vi "GetChimeraResources.vi"(8 "error in (no error)":errorcluster, 11 "Automotive Vision Device selector":refnum<vi>) -> (0 "error out":errorcluster, 1 "Bitfiles":string[](array[string]), 2 "Available input channels on Automotive Camera Vision Devices":string[][](array[string]), 3 "Device Aliases":string[](array[string]))   [LabVIEW 2025]
doc: "Finds all available Automative Vision devices (like PXIe-1486, etc.) , filter them for those what has inputs, gathers all of the input channels, resources, types, and corresponding bitfile."
uses:
  <vilib>/nisyscfg/Filter Mode.ctl
  <vilib>/nisyscfg/nisyscfg.lvlib
  <resource>/objmgr/niflexrioatomicsae.rc
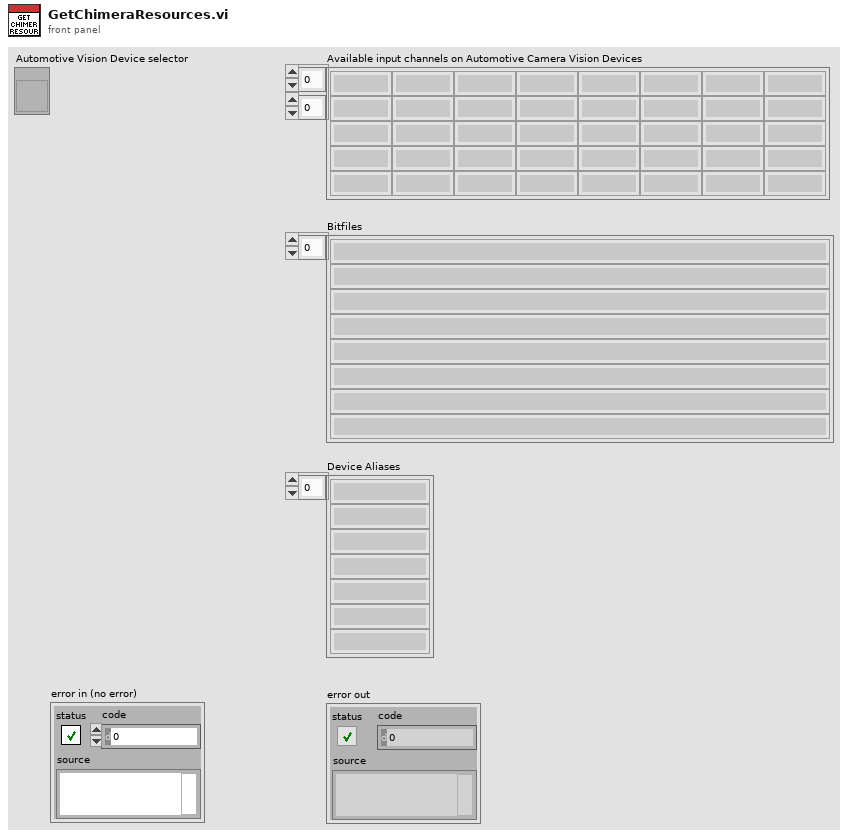
[diagram p1: front panel]
types:
  T1 = typedef "nisyscfg.lvlib/Filter Mode.ctl" = i32
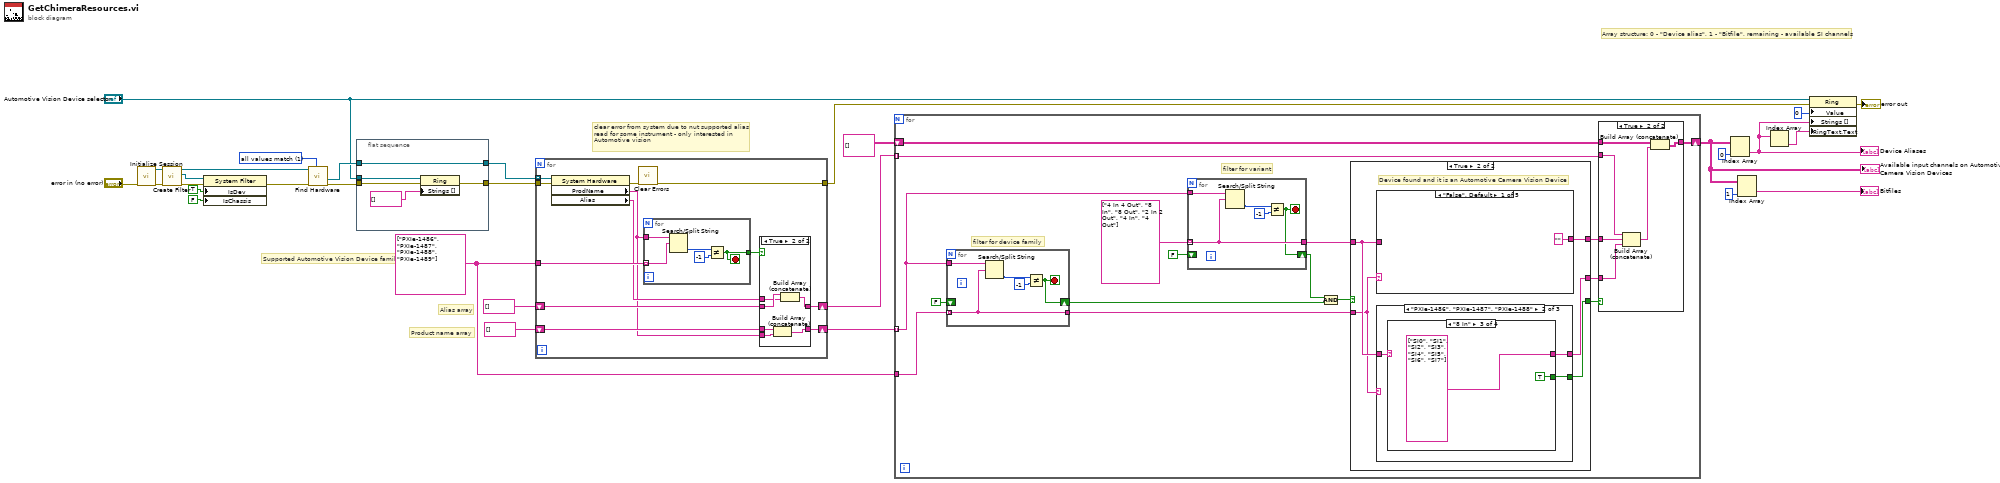
[diagram p0: block diagram]
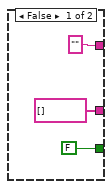
[diagram p3: hidden frame]
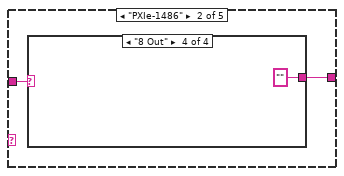
[diagram p4: hidden frame]
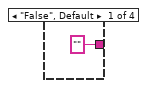
[diagram p5: hidden frame]
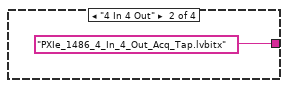
[diagram p6: hidden frame]
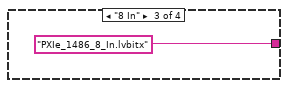
[diagram p7: hidden frame]
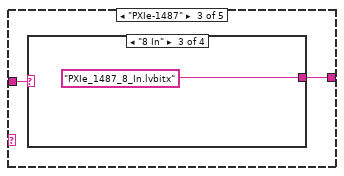
[diagram p8: hidden frame]
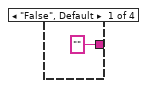
[diagram p9: hidden frame]
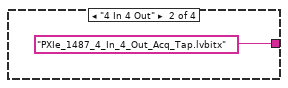
[diagram p10: hidden frame]
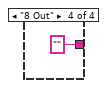
[diagram p11: hidden frame]
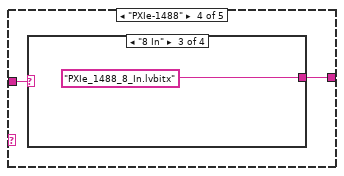
[diagram p12: hidden frame]
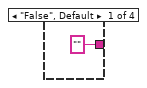
[diagram p13: hidden frame]
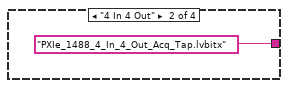
[diagram p14: hidden frame]
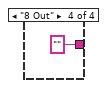
[diagram p15: hidden frame]
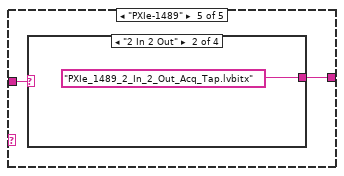
[diagram p16: hidden frame]
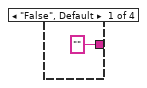
[diagram p17: hidden frame]
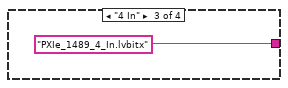
[diagram p18: hidden frame]
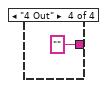
[diagram p19: hidden frame]
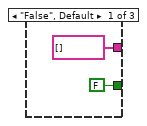
[diagram p20: hidden frame]
diagram:
  w2 = string[] ["PXIe-1486", "PXIe-1487", "PXIe-1488", "PXIe-1489"]
  w18 = T1 1 items=["all values match"=1, "any value matches"=2, "values do not match"=3, "all properties exist"=4] ("Filter Mode (all values match)")
  # "Supported Automotive Vision Device families"
  # "clear error from system due to nut supported alias read for some instrument - only interested in Automotive vision"
  # "Array structure: 0 - \"Device alias\", 1 - \"Bitfile\", remaining - available SI channels"
  # "Product name array"
  # "Alias array"
  n1 = call <vilib>:"Initialize Session.vi"("error in (no error)"="error in (no error)") -> ("error out"=w21:errorcluster, "Session out"=w24:refnum<k21>)  [unwired: 9 in]
  n2 = call <vilib>:"Create Filter.vi"("error in (no error)"=w21, "Session in"=w24) -> ("error out"=w19:errorcluster, "Filter out"=w20:refnum<k20>, "Session out"=w25:refnum<k21>)  [unwired: 7 in]
  n3 = property on="Property Node" class="System Filter"(reference=w20, error in=w19, "IsDev"=TRUE ("Is Chassis"), "IsChassis"=FALSE ("Is Chassis")) -> (error out=w28:errorcluster)  [unwired: 1 out]
  n4 = call <vilib>:"Find Hardware.vi"("Filter Mode (all values match)"=w18, "error in (no error)"=w28, "Session in"=w25) -> ("error out"=w29:errorcluster, "Resources out"=w27:refnum<k20>[])  [unwired: 5 in, 2 out]
  n5 = flat-sequence {
    tunnel: [w35] -> w17
    tunnel: w27 -> [w35]
    tunnel: w29 -> [w34]
    tunnel: [w32] -> w30
    tunnel: "Automotive Vision Device selector" -> [w33]
    frame #0 {
      n6 = property on="Property Node" class="Ring"(reference=w33, error in=w34, "Strings []"=string[] []) -> (error out=w32:errorcluster)  [unwired: 1 out]
    }
  }
  n7 = for {
    tunnel: w17 -> [w46] mode=indexing
    tunnel: w2 -> [w45]
    shift-right: [w44] -> w14
    shift-left: string[] [] -> [w43]
    tunnel: w30 -> [w40]
    tunnel: [w39] -> w5
    shift-right: [w36] -> w15
    shift-left: string[] [] -> [w38]
    n8 = property on="Property Node" class="System Hardware"(reference=w46, error in=w40) -> (error out=w47:errorcluster, "ProdName"=w37:string, "Alias"=w41:string)  [unwired: 1 out]
    n9 = call <vilib>:"Clear Errors.vi"("error in (no error)"=w47) -> ("error out"=w39:errorcluster)  [unwired: 5 in, 1 out]
    n10 = for {
      tunnel: w37 -> [w60]
      tunnel: w45 -> [w59] mode=indexing
      tunnel: [w56] -> w42
      stop <- w56 stop-if-true
      n11 = Search/Split String(string=w60, search string/char (-)=w59) -> (offset of match=w58:i32)  [unwired: 1 in, 2 out]
      n12 = Not Equal?(x=w58, y=-1) -> (x != y?=w56:bool)
    }
    n13 = case shown="True" w42 {
      tunnel: [w49 w54] -> w44
      tunnel: w43 -> [w49 w55]
      tunnel: w41 -> [_ w53]
      tunnel: w38 -> [w48 w52]
      tunnel: w37 -> [_ w51]
      tunnel: [w48 w50] -> w36
      frame False {
      }
      frame True {
        n14 = Build Array (concatenate)(w52, w51) -> (w50:string[])
        n15 = Build Array (concatenate)(w55, w53) -> (w54:string[])
      }
    }
  }
  n16 = for {
    tunnel: w15 -> [w61] mode=indexing
    tunnel: w14 -> [w68] mode=indexing
    shift-right: [w64] -> w9
    shift-left: string[][] [] -> [w63]
    tunnel: w2 -> [w62]
    # "filter for variant"
    # "filter for device family"
    n17 = for {
      tunnel: w61 -> [w93]
      tunnel: w62 -> [w90] mode=indexing
      tunnel: [w90] -> w73
      shift-right: [w89] -> w71
      shift-left: FALSE -> [_]
      stop <- w89 stop-if-true
      n18 = Search/Split String(string=w93, search string/char (-)=w90) -> (offset of match=w91:i32)  [unwired: 1 in, 2 out]
      n19 = Not Equal?(x=w91, y=-1) -> (x != y?=w89:bool)
    }
    n20 = for {
      tunnel: w61 -> [w88]
      tunnel: string[] ["4 In 4 Out", "8 In", "8 Out", "2 In 2 Out", "4 In", "4 Out"] -> [w85] mode=indexing
      tunnel: [w85] -> w69
      shift-right: [w84] -> w72
      shift-left: FALSE -> [_]
      stop <- w84 stop-if-true
      n21 = Search/Split String(string=w88, search string/char (-)=w85) -> (offset of match=w86:i32)  [unwired: 1 in, 2 out]
      n22 = Not Equal?(x=w86, y=-1) -> (x != y?=w84:bool)
    }
    n23 = And(x=w72, y=w71) -> (x .and. y?=w70:bool)
    n24 = case shown="True" w70 {
      tunnel: w73 -> [_ w98]
      tunnel: w69 -> [_ w99]
      tunnel: [string[] [] w101] -> w67
      tunnel: [FALSE w100] -> w66
      tunnel: ["" w97] -> w65
      frame False {
      }
      frame True {
        # "Device found and it is an Automotive Camera Vision Device"
        n25 = case shown="\"PXIe-1486\", \"PXIe-1487\", \"PXIe-1488\"" w98 {
          tunnel: w99 -> [_ w131 w142]
          tunnel: [string[] [] w130 w141] -> w101
          tunnel: [FALSE w129 w140] -> w100
          frame "False", Default {
          }
          frame "PXIe-1486", "PXIe-1487", "PXIe-1488" {
            n26 = case shown="\"8 In\"" w131 {
              tunnel: [string[] [] string[] ["SI0", "SI1", "SI2", "SI3"] string[] ["SI0", "SI1", "SI2", "SI3", "SI4", "SI5", "SI6", "SI7"] string[] []] -> w130
              tunnel: [FALSE TRUE TRUE FALSE] -> w129
              frame "False", Default {
              }
              frame "4 In 4 Out" {
              }
              frame "8 In" {
              }
              frame "8 Out" {
              }
            }
          }
          frame "PXIe-1489" {
            n27 = case shown="\"False\", Default" w142 {
              tunnel: [string[] [] string[] ["SI0", "SI1"] string[] ["SI0", "SI1", "SI2", "SI3"] string[] []] -> w141
              tunnel: [FALSE TRUE TRUE FALSE] -> w140
              frame "False", Default {
              }
              frame "2 In 2 Out" {
              }
              frame "4 In" {
              }
              frame "4 Out" {
              }
            }
          }
        }
        n28 = case shown="\"False\", Default" w98 {
          tunnel: ["" w104 w110 w116 w122] -> w97
          tunnel: w99 -> [_ w103 w109 w115 w121]
          frame "False", Default {
          }
          frame "PXIe-1486" {
            n29 = case shown="\"8 Out\"" w103 {
              tunnel: ["" "PXIe_1486_4_In_4_Out_Acq_Tap.lvbitx" "PXIe_1486_8_In.lvbitx" ""] -> w104
              frame "False", Default {
              }
              frame "4 In 4 Out" {
              }
              frame "8 In" {
              }
              frame "8 Out" {
              }
            }
          }
          frame "PXIe-1487" {
            n30 = case shown="\"8 In\"" w109 {
              tunnel: ["" "PXIe_1487_4_In_4_Out_Acq_Tap.lvbitx" "PXIe_1487_8_In.lvbitx" ""] -> w110
              frame "False", Default {
              }
              frame "4 In 4 Out" {
              }
              frame "8 In" {
              }
              frame "8 Out" {
              }
            }
          }
          frame "PXIe-1488" {
            n31 = case shown="\"8 In\"" w115 {
              tunnel: ["" "PXIe_1488_4_In_4_Out_Acq_Tap.lvbitx" "PXIe_1488_8_In.lvbitx" ""] -> w116
              frame "False", Default {
              }
              frame "4 In 4 Out" {
              }
              frame "8 In" {
              }
              frame "8 Out" {
              }
            }
          }
          frame "PXIe-1489" {
            n32 = case shown="\"2 In 2 Out\"" w121 {
              tunnel: ["" "PXIe_1489_2_In_2_Out_Acq_Tap.lvbitx" "PXIe_1489_4_In.lvbitx" ""] -> w122
              frame "False", Default {
              }
              frame "2 In 2 Out" {
              }
              frame "4 In" {
              }
              frame "4 Out" {
              }
            }
          }
        }
      }
    }
    n33 = case shown="True" w66 {
      tunnel: w68 -> [_ w83]
      tunnel: w67 -> [_ w81]
      tunnel: w65 -> [_ w82]
      tunnel: [w77 w79] -> w64
      tunnel: w63 -> [w77 w80]
      frame False {
      }
      frame True {
        n34 = Build Array (concatenate)(w83, w82, w81) -> (w78:string[])
        n35 = Build Array (concatenate)(w80, w78) -> (w79:string[][])
      }
    }
  }
  "Available input channels on Automotive Camera Vision Devices" <- w9
  n36 = Index Array(array=w9, index (col)=0 ("disabled index (col)")) -> (element=w6:string[])  [unwired: 1 in]
  "Device Aliases" <- w6
  n37 = Index Array(array=w9, index (col)=1 ("disabled index (col)")) -> (element=→"Bitfiles":string[])  [unwired: 1 in]
  n38 = Index Array(array=w6) -> (element=w13:string)  [unwired: 1 in]
  n39 = property on="Property Node" class="Ring"(reference="Automotive Vision Device selector", error in=w5, "Value"=0, "Strings []"=w6, "RingText.Text"=w13) -> (error out=→"error out":errorcluster)  [unwired: 1 out]
